vi "Audio File Refnum To Value.vi"(11 "Audio File Refnum":T1) -> (3 "Refnum Value":i32)   [LabVIEW 2020, in "G-Audio.lvlib"]
uses:
  G-Audio.lvlib
  Controls/Audio File Refnum.ctl
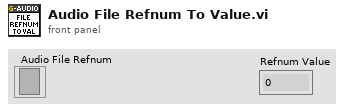
[diagram p1: front panel]
types:
  T1 = typedef "G-Audio.lvlib/Audio File Refnum.ctl" = refnum<file>
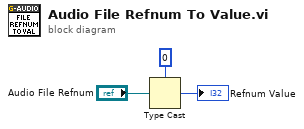
[diagram p0: block diagram]
diagram:
  n1 = Type Cast(type=0, x="Audio File Refnum") -> (*(type *) &x=→"Refnum Value":i32)
